vi "Math-updater-w--for-same-SpVar-names-28012016.vi"(0 "Sp_Id_Arr":string[](array[string]), 1 "Math Expressions":string[](array[string]), 2 "Pr_Id_Arr":string[](array[string]), 3 "LP-Cnt_4_Reac":string[](array[string]), 4 "LP_IDs":string[](array[string])) -> (5 "New Total Pr IDs":string[](array[string]), 6 "Math-w/-ch-VarID":string[](array[string]))   [LabVIEW 2014]
doc: "This VI checks if the variable and species name are same. If they are, then the math is updated with the new variable name in order to distinguish their value."
panel:
  out "j":i32
  out "k":i32
  out "New Pr IDs":string[](array[string])
  out "New LP IDs":string[](array[string])
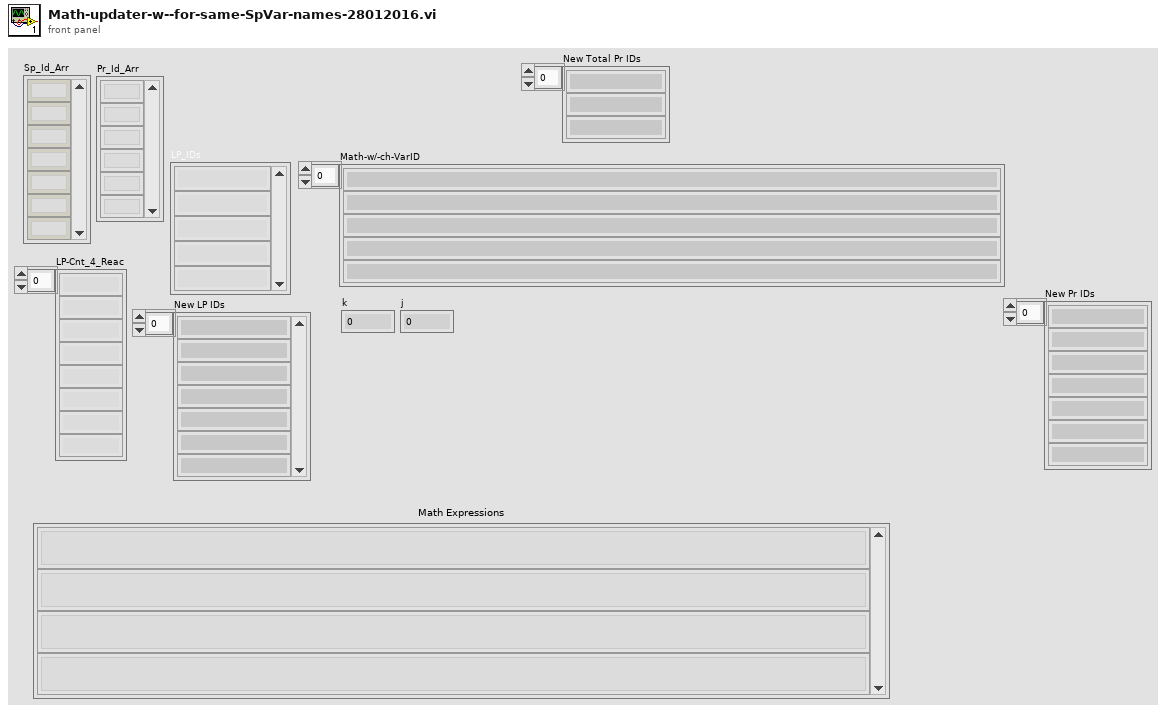
[diagram p1: front panel]
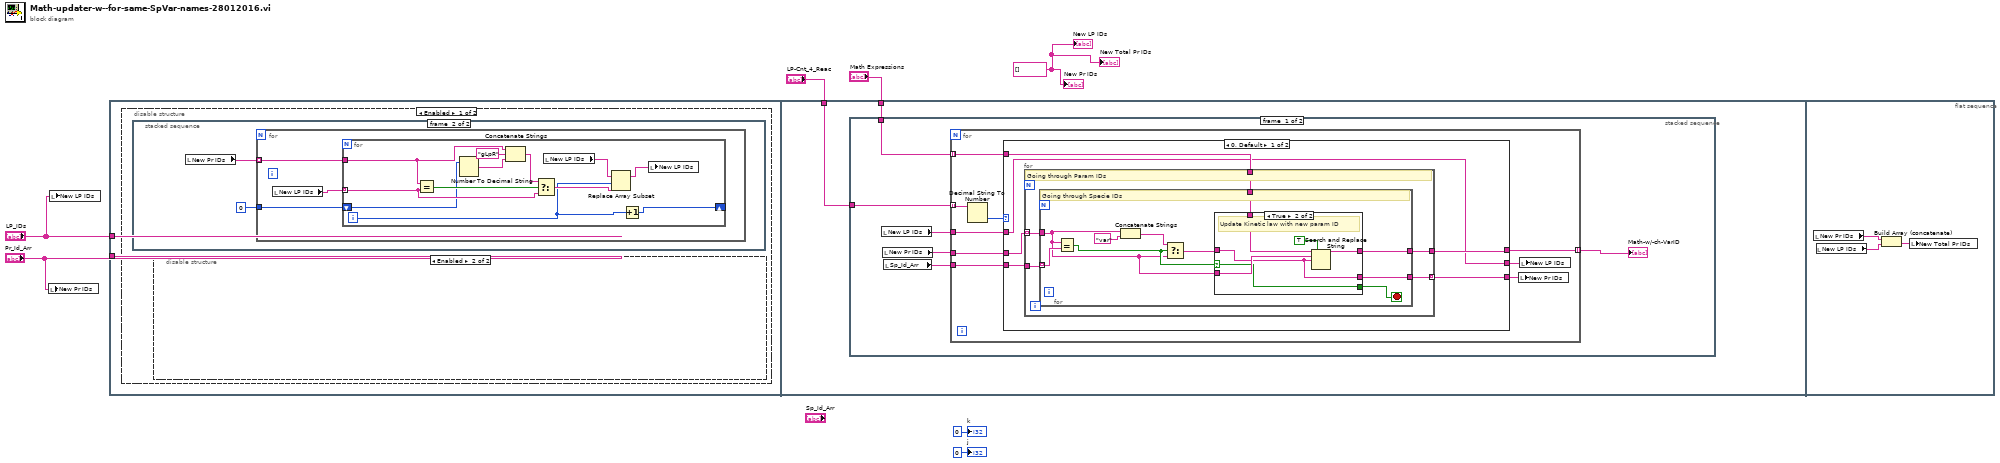
[diagram p0: block diagram]
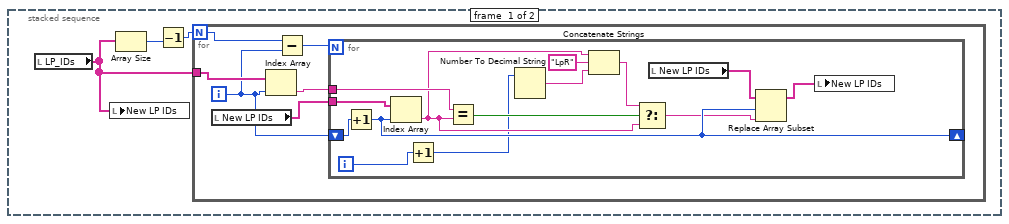
[diagram p2: hidden frame]
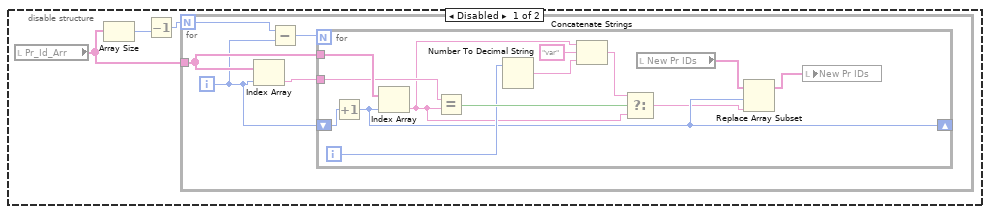
[diagram p3: hidden frame]
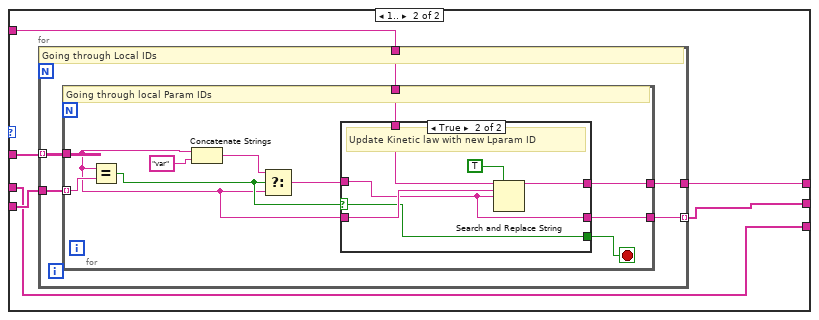
[diagram p6: hidden frame]
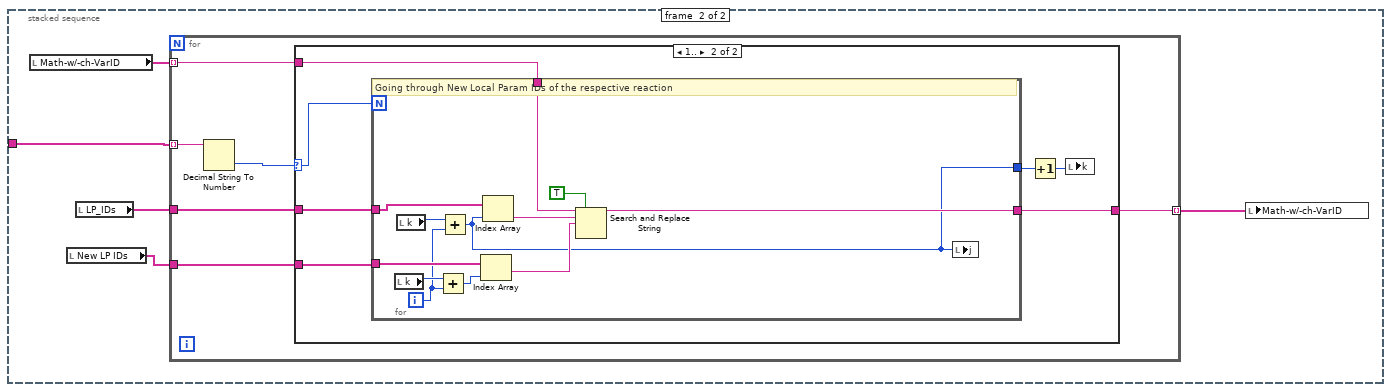
[diagram p8: hidden frame]
diagram:
  w7 = string[] [] ("New LP IDs")
  n1 = local write "New Pr IDs"("Pr_Id_Arr") -> ()
  n2 = local write "New LP IDs"("LP_IDs") -> ()
  n3 = flat-sequence {
    tunnel: "Pr_Id_Arr" -> [_]
    tunnel: "LP_IDs" -> [_]
    tunnel: "Math Expressions" -> [w70]
    tunnel: "LP-Cnt_4_Reac" -> [w69]
    frame #0 {
      n4 = disable-structure shown="Enabled" {
        frame Enabled {
          n5 = stacked-sequence {
            frame #0 {
              n6 = local read "LP_IDs"() -> (w8:string[])
              n7 = local write "New LP IDs"(w8) -> ()
              n8 = Array Size(array=w8) -> (size(s)=w10:i32)
              n9 = Decrement(x=w10) -> (x-1=w9:i32)
              n10 = for {
                N: w9 -> [w16]
                tunnel: w8 -> [w14]
                i -> [w12]
                n11 = local read "New LP IDs"() -> (w11:string[])
                n12 = Index Array(array=w14, index=w12) -> (element=w13:string)
                n13 = Subtract(x=w16, y=w12) -> (x-y=w15:i32)
                n14 = for {
                  N: w15 -> [_]
                  tunnel: w13 -> [w30]
                  shift-right: [w22] -> _
                  shift-left: w12 -> [w28]
                  tunnel: w11 -> [w17]
                  i -> [w19]
                  n15 = Increment(x=w28) -> (x+1=w22:i32)
                  n16 = Index Array(array=w17, index=w22) -> (element=w24:string)
                  n17 = Increment(x=w19) -> (x+1=w18:i32)
                  n18 = Equal?(x=w30, y=w24) -> (x = y?=w29:bool)
                  n19 = Number To Decimal String(number=w18) -> (decimal integer string=w25:string)  [unwired: 1 in]
                  n20 = Concatenate Strings(w24, "LpR" ("string"), w25) -> (w27:string)
                  n21 = Select(t=w27, s=w29, f=w24) -> (s? t:f=w21:string)
                  n22 = local read "New LP IDs"() -> (w23:string[])
                  n23 = Replace Array Subset(array=w23, new element=w21, index=w22) -> (w20:string[])
                  n24 = local write "New LP IDs"(w20) -> ()
                }
              }
            }
            frame #1 {
              n25 = local read "New Pr IDs"() -> (w32:string[])
              n26 = for {
                tunnel: w32 -> [w35] mode=indexing
                tunnel: 0 -> [w33]
                n27 = local read "New LP IDs"() -> (w34:string[])
                n28 = for {
                  tunnel: w35 -> [w40]
                  tunnel: w34 -> [w39] mode=indexing
                  shift-right: [w36] -> _
                  shift-left: w33 -> [w38]
                  i -> [w37]
                  n29 = Equal?(x=w40, y=w39) -> (x = y?=w47:bool)
                  n30 = Number To Decimal String(number=w38) -> (decimal integer string=w44:string)  [unwired: 1 in]
                  n31 = Concatenate Strings(w40, "gLpR" ("string"), w44) -> (w46:string)
                  n32 = Select(t=w46, s=w47, f=w39) -> (s? t:f=w42:string)
                  n33 = local read "New LP IDs"() -> (w43:string[])
                  n34 = Replace Array Subset(array=w43, new element=w42, index=w37) -> (w41:string[])
                  n35 = Increment(x=w37) -> (x+1=w36:i32)
                  n36 = local write "New LP IDs"(w41) -> ()
                }
              }
            }
          }
          n37 = disable-structure shown="Enabled" {
            frame Disabled {
              n38 = local read "Pr_Id_Arr"() -> (w48:string[])
              n39 = Array Size(array=w48) -> (size(s)=w49:i32)
              n40 = Decrement(x=w49) -> (x-1=w50:i32)
              n41 = for {
                N: w50 -> [w55]
                tunnel: w48 -> [w53]
                i -> [w51]
                n42 = Index Array(array=w53, index=w51) -> (element=w52:string)
                n43 = Subtract(x=w55, y=w51) -> (x-y=w54:i32)
                n44 = for {
                  N: w54 -> [_]
                  tunnel: w53 -> [w68]
                  tunnel: w52 -> [w67]
                  shift-right: [w58] -> _
                  shift-left: w51 -> [w65]
                  i -> [w61]
                  n45 = Increment(x=w65) -> (x+1=w58:i32)
                  n46 = Index Array(array=w68, index=w58) -> (element=w60:string)
                  n47 = Equal?(x=w67, y=w60) -> (x = y?=w66:bool)
                  n48 = Number To Decimal String(number=w61) -> (decimal integer string=w62:string)  [unwired: 1 in]
                  n49 = Concatenate Strings(w60, "var" ("string"), w62) -> (w64:string)
                  n50 = Select(t=w64, s=w66, f=w60) -> (s? t:f=w57:string)
                  n51 = local read "New Pr IDs"() -> (w59:string[])
                  n52 = Replace Array Subset(array=w59, new element=w57, index=w58) -> (w56:string[])
                  n53 = local write "New Pr IDs"(w56) -> ()
                }
              }
            }
            frame Enabled {
            }
          }
        }
        frame Disabled {
        }
      }
    }
    frame #1 {
      n54 = stacked-sequence {
        tunnel: w70 -> [w76 _]
        tunnel: w69 -> [w75 w150]
        frame #0 {
          n55 = local read "New LP IDs"() -> (w74:string[])
          n56 = local read "New Pr IDs"() -> (w73:string[])
          n57 = local read "Sp_Id_Arr"() -> (w72:string[])
          n58 = for {
            tunnel: w76 -> [w81] mode=indexing
            tunnel: w75 -> [w85] mode=indexing
            tunnel: w74 -> [w83]
            tunnel: w72 -> [w82]
            tunnel: [w80] -> w71 mode=indexing
            tunnel: w73 -> [w79]
            n59 = Decimal String To Number(string=w85) -> (number=w84:i32)  [unwired: 2 in, 1 out]
            n60 = case shown="0, Default" w84 {
              tunnel: w83 -> [w86 w121]
              tunnel: w82 -> [w89 w120]
              tunnel: w81 -> [w90 w119]
              tunnel: [w91 w118] -> w80
              tunnel: w79 -> [w88 w117]
              tunnel: [w87 w117] -> w78
              tunnel: [w86 w116] -> w77
              frame 0, Default {
                n61 = for {
                  tunnel: w88 -> [w96] mode=indexing
                  tunnel: w89 -> [w95]
                  tunnel: w90 -> [w94]
                  tunnel: [w93] -> w91
                  tunnel: [w92] -> w87 mode=indexing
                  # "Going through Param IDs"
                  n62 = for {
                    tunnel: w96 -> [w100]
                    tunnel: w95 -> [w106] mode=indexing
                    tunnel: w94 -> [w101]
                    tunnel: [w99] -> w93
                    tunnel: [w97] -> w92
                    stop <- w98 stop-if-true
                    # "Going through Specie IDs"
                    n63 = Equal?(x=w100, y=w106) -> (x = y?=w103:bool)
                    n64 = Concatenate Strings(w100, "var") -> (w105:string)
                    n65 = Select(t=w105, s=w103, f=w100) -> (s? t:f=w102:string)
                    n66 = case shown="True" w103 {
                      selector: w103 -> [w108 w111]
                      tunnel: w102 -> [_ w110]
                      tunnel: w101 -> [w109 w114]
                      tunnel: w100 -> [w107 w113]
                      tunnel: [w109 w112] -> w99
                      tunnel: [w108 w111] -> w98
                      tunnel: [w107 w110] -> w97
                      frame False {
                      }
                      frame True {
                        # "Update Kinetic law with new param ID"
                        n67 = Search and Replace String(replace all?=TRUE ("replace all? (F)"), input string=w114, search string=w113, replace string=w110) -> (result string=w112:string)  [unwired: 4 in, 3 out]
                      }
                    }
                  }
                }
              }
              frame 1.. {
                n68 = for {
                  tunnel: w121 -> [w126] mode=indexing
                  tunnel: w120 -> [w125]
                  tunnel: w119 -> [w124]
                  tunnel: [w123] -> w118
                  tunnel: [w122] -> w116 mode=indexing
                  # "Going through Local IDs"
                  n69 = for {
                    tunnel: w126 -> [w130]
                    tunnel: w125 -> [w136] mode=indexing
                    tunnel: w124 -> [w131]
                    tunnel: [w129] -> w123
                    tunnel: [w127] -> w122
                    stop <- w128 stop-if-true
                    # "Going through local Param IDs"
                    n70 = Equal?(x=w130, y=w136) -> (x = y?=w133:bool)
                    n71 = Concatenate Strings(w130, "var") -> (w135:string)
                    n72 = Select(t=w135, s=w133, f=w130) -> (s? t:f=w132:string)
                    n73 = case shown="True" w133 {
                      selector: w133 -> [w138 w141]
                      tunnel: w132 -> [_ w140]
                      tunnel: w131 -> [w139 w144]
                      tunnel: w130 -> [w137 w143]
                      tunnel: [w139 w142] -> w129
                      tunnel: [w138 w141] -> w128
                      tunnel: [w137 w140] -> w127
                      frame False {
                      }
                      frame True {
                        # "Update Kinetic law with new Lparam ID"
                        n74 = Search and Replace String(replace all?=TRUE ("replace all? (F)"), input string=w144, search string=w143, replace string=w140) -> (result string=w142:string)  [unwired: 4 in, 3 out]
                      }
                    }
                  }
                }
              }
            }
            n75 = local write "New Pr IDs"(w78) -> ()
            n76 = local write "New LP IDs"(w77) -> ()
          }
          "Math-w/-ch-VarID" <- w71
        }
        frame #1 {
          n77 = local read "Math-w/-ch-VarID"() -> (w147:string[])
          n78 = local read "New LP IDs"() -> (w148:string[])
          n79 = local read "LP_IDs"() -> (w146:string[])
          n80 = for {
            tunnel: w147 -> [w153] mode=indexing
            tunnel: w150 -> [w156] mode=indexing
            tunnel: w148 -> [w154]
            tunnel: [w152] -> w149 mode=indexing
            tunnel: w146 -> [w151]
            n81 = Decimal String To Number(string=w156) -> (number=w155:i32)  [unwired: 2 in, 1 out]
            n82 = case shown="1.." w155 {
              selector: w155 -> [_ w160]
              tunnel: w154 -> [_ w164]
              tunnel: w153 -> [w157 w163]
              tunnel: [w157 w162] -> w152
              tunnel: w151 -> [_ w161]
              frame 0, Default {
              }
              frame 1.. {
                n83 = for {
                  N: w160 -> [_]
                  tunnel: w164 -> [w173]
                  tunnel: w163 -> [w176]
                  tunnel: [w175] -> w162
                  tunnel: w161 -> [w169]
                  tunnel: [w165] -> w159
                  i -> [w168]
                  # "Going through New Local Param IDs of the respective reaction"
                  n84 = local read "k"() -> (w172:i32)
                  n85 = local read "k"() -> (w170:i32)
                  n86 = Add(x=w172, y=w168) -> (x+y=w171:i32)
                  n87 = Add(x=w170, y=w168) -> (x+y=w165:i32)
                  n88 = Index Array(array=w173, index=w171) -> (element=w166:string)
                  n89 = Index Array(array=w169, index=w165) -> (element=w167:string)
                  n90 = Search and Replace String(replace all?=TRUE ("replace all? (F)"), input string=w176, search string=w167, replace string=w166) -> (result string=w175:string)  [unwired: 4 in, 3 out]
                  n91 = local write "j"(w165) -> ()
                }
                n92 = Increment(x=w159) -> (x+1=w158:i32)
                n93 = local write "k"(w158) -> ()
              }
            }
          }
          n94 = local write "Math-w/-ch-VarID"(w149) -> ()
        }
      }
    }
    frame #2 {
      n95 = local read "New Pr IDs"() -> (w178:string[])
      n96 = local read "New LP IDs"() -> (w179:string[])
      n97 = Build Array (concatenate)(w178, w179) -> (w177:string[])
      n98 = local write "New Total Pr IDs"(w177) -> ()
    }
  }
  "New LP IDs" <- w7
  "New Pr IDs" <- w7
  "New Total Pr IDs" <- w7
  "k" <- 0 ("LP Off")
  "j" <- 0 ("LP Off")
